vi "ingest_journalJson.vi"(6 "channel":string, 8 "error in":errorcluster, 9 "Target":refnum<class "target.lvclass">, 10 "Source":refnum<class "source.lvclass">, 11 "Nominal Client in":refnum<class "Nominal Client.lvclass">) -> (0 "error out":errorcluster, 1 "datasetRid":string, 2 "datasetFileId":string, 3 "Nominal Client out":refnum<class "Nominal Client.lvclass">)   [LabVIEW 2020, in "Nominal Client.lvclass"]
doc: "Triggers an ingest job, allowing either creating a new dataset or uploading to an existing one. This endpoint is meant to supersede all other ingestion endpoints as their functionality gets migrated to this one."
uses:
  Nominal Client.lvclass
  datasources/target/target.lvclass
  datasources/source/source.lvclass
  Nominal Client.lvclass/Nominal Client.ctl
  datasources/target/target.lvclass/target.ctl
  ac599124-47d5-44f8-8944-41970eb09d00.vi
  c811998a-e5cf-4f6e-88ed-9ebe04757b7f.vi
  datasources/target/workspace.set.vi
  <vilib>/JDP Science/JSONtext/Variant to JSON Text.vi
  <vilib>/JDP Science/JSONtext/support/Format JSON Object.vi
  <vilib>/JDP Science/JSONtext/JSON text to Variant.vi
  <vilib>/JDP Science/JSONtext/LVClass Serializer/JSONtext LVClass Serializer.lvclass
  <vilib>/JDP Science/JSONtext/JSONtext.lvlib
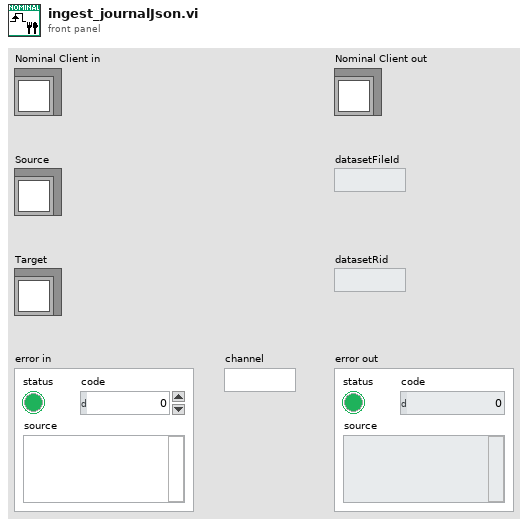
[diagram p1: front panel]
types:
  T1 = cluster{"type":string, "dataset":cluster{"datasetFileId":string, "datasetRid":string}}
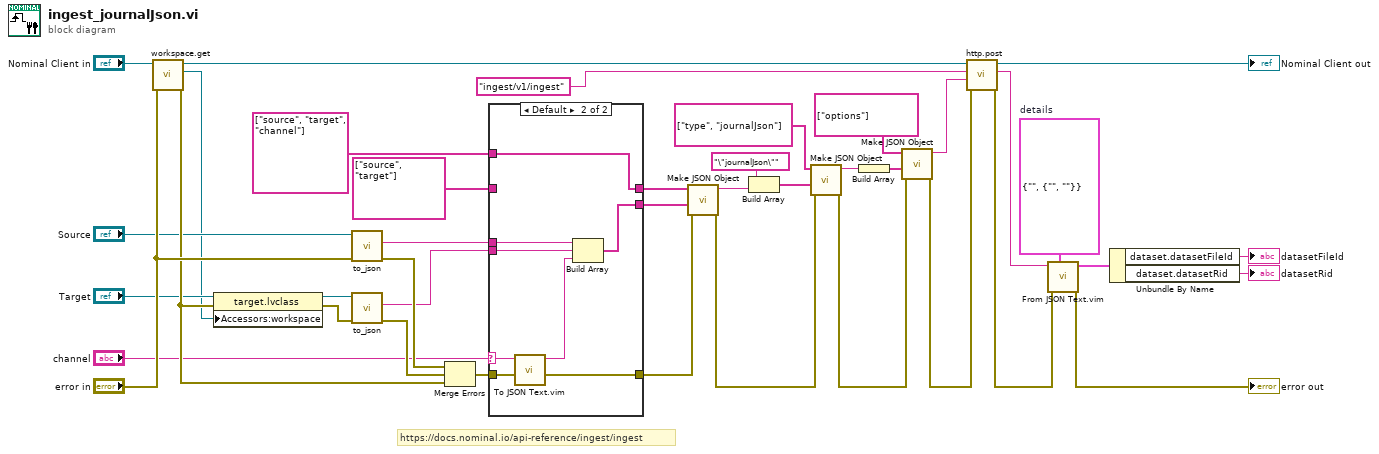
[diagram p0: block diagram]
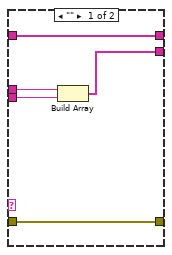
[diagram p2: hidden frame]
diagram:
  w13 = T1 {"type"="", "dataset"={"datasetFileId"="", "datasetRid"=""}}  # details
  # "https://docs.nominal.io/api-reference/ingest/ingest"
  n1 = call "workspace.get.vi"("error in"="error in", "Nominal Client in"="Nominal Client in") -> ("error out"=w29:errorcluster, "workspace"=w19:refnum<class "workspace.lvclass">, "Nominal Client out"=w31:refnum<class "Nominal Client.lvclass">)  [unwired: 7 in]
  n2 = property class="target.lvclass"(reference="Target", error in=w29, "Accessors:workspace"=w19) -> (reference out=w33:refnum<class "target.lvclass">, error out=w34:errorcluster)
  n3 = call-dynamic "to_json.vi"("error in"="error in", "source in"="Source") -> ("error out"=w37:errorcluster, "json"=w38:string)  [unwired: 6 in, 2 out]
  n4 = call-dynamic "to_json.vi"("error in"=w34, "target in"=w33) -> ("error out"=w36:errorcluster, "json"=w35:string)  [unwired: 6 in, 2 out]
  n5 = Merge Errors(w37, w36, w29) -> (w24:errorcluster)
  n6 = case shown="Default" "channel" {
    selector: "channel" -> [_ w50]
    tunnel: w38 -> [w45 w53]
    tunnel: w35 -> [w44 w52]
    tunnel: [w43 w49] -> w28
    tunnel: string[] ["source", "target", "channel"] ("Path") -> [_ w48]
    tunnel: [w42 w48] -> w26
    tunnel: string[] ["source", "target"] ("Path") -> [w42 _]
    tunnel: w24 -> [w41 w47]
    tunnel: [w41 w46] -> w23
    frame "" {
      n7 = Build Array(w45, w44) -> (w43:string[])
    }
    frame Default {
      n8 = call "To JSON Text.vim"("error in (no error)"=w47, "Anything"=w50) -> ("error out"=w46:errorcluster, "<JSON>"=w51:string)  [unwired: 8 in]
      n9 = Build Array(w53, w52, w51) -> (w49:string[])
    }
  }
  n10 = call <vilib>:"Make JSON Object.vi"("error in (no error)"=w23, "JSON Items"=w28, "Item Names"=w26) -> ("error out"=w14:errorcluster, "<JSON>"=w15:string)  [unwired: 7 in]
  n11 = Build Array("\"journalJson\"" ("JSON"), w15) -> (w17:string[])
  n12 = call <vilib>:"Make JSON Object.vi"("error in (no error)"=w14, "JSON Items"=w17, "Item Names"=string[] ["type", "journalJson"] ("JSON")) -> ("error out"=w2:errorcluster, "<JSON>"=w6:string)  [unwired: 7 in]
  n13 = Build Array(w6) -> (w5:string[])
  n14 = call <vilib>:"Make JSON Object.vi"("error in (no error)"=w2, "JSON Items"=w5, "Item Names"=string[] ["options"] ("JSON")) -> ("error out"=w1:errorcluster, "<JSON>"=w3:string)  [unwired: 7 in]
  n15 = call "http.post.vi"("error in"=w1, "Request body"=w3, "Path"="ingest/v1/ingest", "Nominal Client in"=w31) -> ("error out"=w8:errorcluster, "Response"=w9:string, "Nominal Client out"=→"Nominal Client out":refnum<class "Nominal Client.lvclass">)  [unwired: 4 in, 1 out]
  n16 = call "From JSON Text.vim"("Data Type and Default Value"=w13, "error in (no error)"=w8, "JSON"=w9) -> ("error out"=→"error out":errorcluster, "Data out"=w12:T1)  [unwired: 7 in]
  n17 = Unbundle By Name(w12) -> ("dataset.datasetFileId"=→"datasetFileId":string, "dataset.datasetRid"=→"datasetRid":string)
